vi "local_variable.vi"() -> ()   [LabVIEW 2020]
panel:
  out "Waveform Chart":dbl(graph)
  in  "Tab Control":enum32{"Page 2"}(tab)
  in  "Initial Value":dbl
  in  "value":bool
  in  "Final Value":dbl
  out "Current Result":dbl
  out "loop no":i32
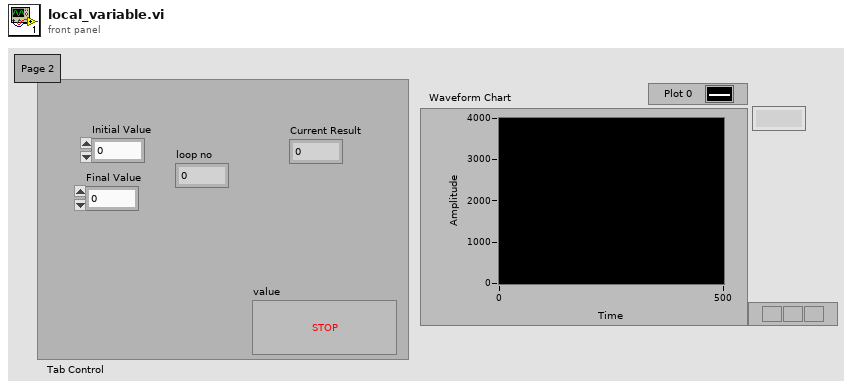
[diagram p1: front panel]
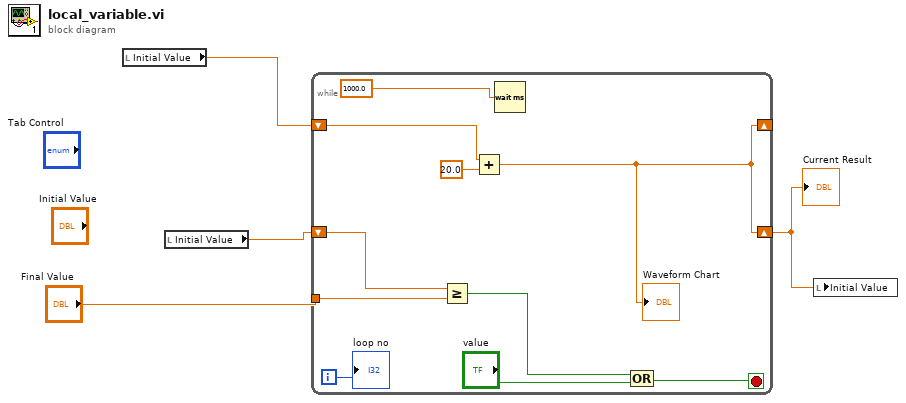
[diagram p0: block diagram]
diagram:
  n1 = local read "Initial Value"() -> (w2:dbl)
  n2 = local read "Initial Value"() -> (w3:dbl)
  n3 = while {
    shift-right: [w8] -> w1
    shift-left: w3 -> [w11]
    tunnel: "Final Value" -> [w9]
    shift-right: [w8] -> _
    shift-left: w2 -> [w5]
    i -> [w7]
    stop <- w14 stop-if-true
    n4 = Greater Or Equal?(x=w11, y=w9) -> (x >= y?=w13:bool)
    n5 = Add(x=w5, y=20.0) -> (x+y=w8:dbl)
    "Waveform Chart" <- w8
    n6 = Wait (ms)(milliseconds to wait=1000.0 ("Initial Value")) -> ()  [unwired: 1 out]
    n7 = Compound Arithmetic op=OR(w13, "value") -> (w14:bool)
    "loop no" <- w7
  }
  "Current Result" <- w1
  n8 = local write "Initial Value"(w1) -> ()
